vi "Parser-iterate.vi"() -> (0 "Statusbyte":i32)   [LabVIEW 2019]
uses:
  Controls/Parser-data.ctl
panel:
  in  "MIDI Parse Data In":T1={"MIDI-Bytes In"=[145, 60, 100], "MIDI Tag"=[], "MIDI Parsed Data"=[], "Iteration"=0, "Error?"=[], "Running States"=[], "Running Statusbyte"=0, "Running StatusString"="", "Third Byte Flag"=FALSE, "Current Byte"=0, "Sysex"="", "Expect Databyte"=FALSE} {"Current Byte" format="%.0x"; "Running Statusbyte" format="%.0x"; "MIDI-Bytes In" format="%.0x"}
  out "MIDI Parse Data Out":T1={"MIDI-Bytes In"=[145, 60, 100], "MIDI Tag"=[], "MIDI Parsed Data"=[], "Iteration"=0, "Error?"=[], "Running States"=[], "Running Statusbyte"=0, "Running StatusString"="", "Third Byte Flag"=FALSE, "Current Byte"=0, "Sysex"="", "Expect Databyte"=FALSE} {"Current Byte" format="%.0x"; "Running Statusbyte" format="%.0x"; "MIDI-Bytes In" format="%.0x"}
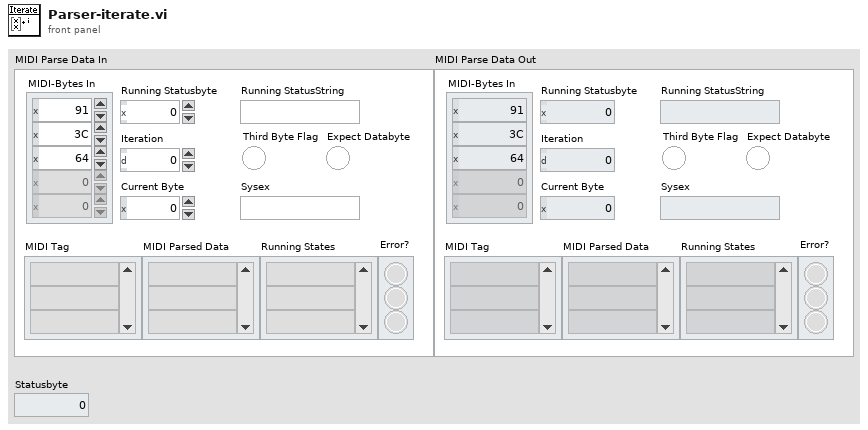
[diagram p1: front panel]
types:
  T1 = typedef "Parser-data.ctl" = cluster{"MIDI-Bytes In":u8[], "MIDI Tag":string[], "MIDI Parsed Data":string[], "Iteration":i32, "Error?":bool[], "Running States":string[], "Running Statusbyte":u8, "Running StatusString":string, "Third Byte Flag":bool, "Current Byte":u8, "Sysex":string, "Expect Databyte":bool}
  T2 = cluster{"MIDI-Bytes In":i32[], "MIDI Tag":string[], "MIDI Parsed Data":string[], "Iteration":i32, "Error?":bool[], "Running State":string[]}
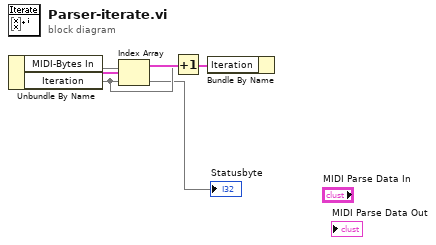
[diagram p0: block diagram]
diagram:
  n1 = Unbundle By Name() -> (w5:T2, "MIDI-Bytes In"=w1, "Iteration"=w4)
  n2 = Index Array(array=w1, index=w4) -> (element=→"Statusbyte")
  n3 = Increment(x=w4) -> (x+1=w3:dbl)
  n4 = Bundle By Name(cluster=w5, "Iteration"=w3) -> (w6:cluster{})
